vi "Script New Module.vi"(0 "Module Name":string, 1 "Project":refnum<vi>, 5 "Module Type":u16, 7 "ModuleType(String)":string, 9 "Module Save Path":path, 11 "error in (no error)":errorcluster, 12 "Line 1 text":string="MyModule") -> (4 "ModulePath(lvlib)":path, 15 "error out":errorcluster)   [LabVIEW 2014, in "DQMH_API.lvclass"]
uses:
  <resource>/Framework/Providers/Open_GDS/UML/DQMH_API_class/DQMH_API.lvclass
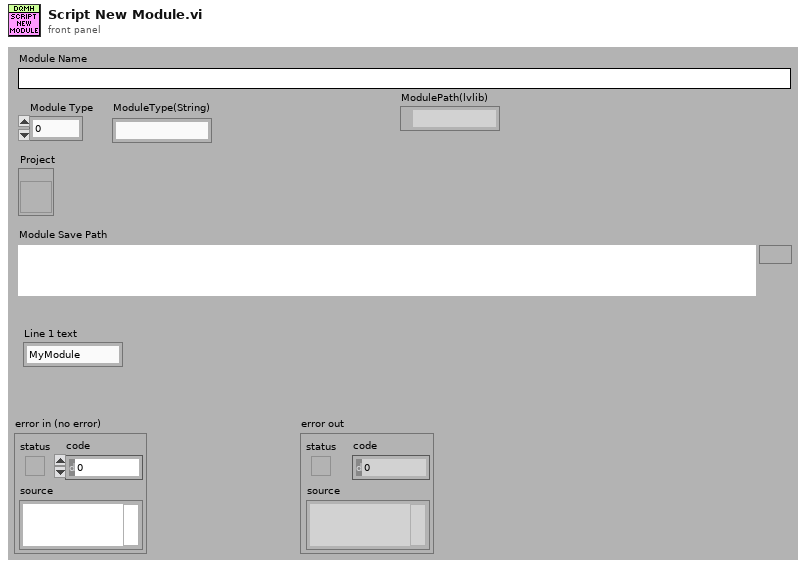
[diagram p1: front panel]
types:
  T1 = typedef "DQMH_API.lvclass/ObjectAttributes.ctl" = cluster{"Get Module Type Info":refnum<vi>, "Script New Module":refnum<vi>, "Script New Event":refnum<vi>}
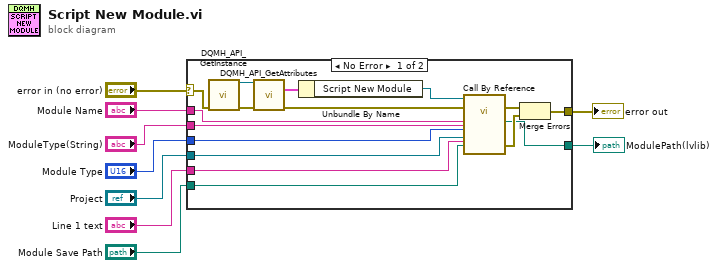
[diagram p0: block diagram]
diagram:
  n1 = case shown="No Error" "error in (no error)" {
    selector: "error in (no error)" -> [w23 w26]
    tunnel: [w18 w26] -> w8
    tunnel: "ModuleType(String)" -> [w16 _]
    tunnel: "Module Name" -> [w15 _]
    tunnel: "Module Type" -> [w14 _]
    tunnel: "Project" -> [w13 _]
    tunnel: "Module Save Path" -> [w12 _]
    tunnel: "Line 1 text" -> [w11 _]
    tunnel: [w10 _] -> w1
    frame No Error {
      n2 = call <resource>:"DQMH_API_GetInstance.vi"("error in (no error)"=w23) -> ("reference out"=w24:refnum<class "DQMH_API.lvclass">, "error out"=w22:errorcluster)  [unwired: 10 in, 3 out]
      n3 = call <resource>:"DQMH_API_GetAttributes.vi"("reference in"=w24, "error in (no error)"=w22) -> ("Data"=w25:T1, "error out"=w20:errorcluster)  [unwired: 10 in, 2 out]
      n4 = Unbundle By Name(w25) -> ("Script New Module"=w21:refnum<vi>)
      n5 = call-by-ref "?"(reference=w21, error in=w20, "Line 1 text"=w11, "ModuleType(String)"=w16, "Module Save Path"=w12, "Project"=w13, "Module Type"=w14, "Module Name"=w15) -> (error out=w19:errorcluster, 0:"error out"=w17:errorcluster, "ModulePath(lvlib)"=w10:path)  [unwired: 4 in, 1 out]
      n6 = Merge Errors(w19, w17) -> (w18:errorcluster)
    }
    frame Error {
    }
  }
  "error out" <- w8
  "ModulePath(lvlib)" <- w1
